vi "UpdateDLLx64.vi"() -> (0 "error out":errorcluster)   [LabVIEW 2017]
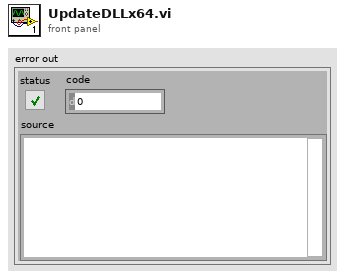
[diagram p1: front panel]
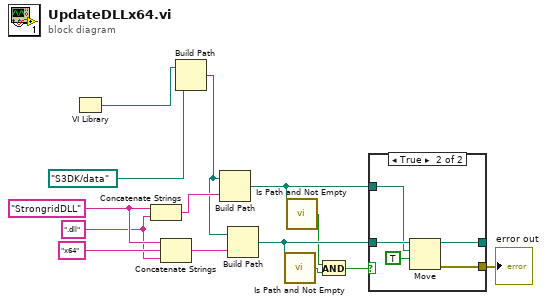
[diagram p0: block diagram]
diagram:
  w12 = ".dll" ("name or relative path")
  w14 = "StrongridDLL" ("name or relative path")
  n1 = VI Library() -> (path=w3:path)
  n2 = Concatenate Strings(w14, w12) -> (w11:string)
  n3 = Concatenate Strings(w14, "x64" ("name or relative path"), w12) -> (w10:string)
  n4 = Build Path(base path=w3, name or relative path=path "S3DK/data") -> (appended path=w1:path)
  n5 = Build Path(base path=w1, name or relative path=w11) -> (appended path=w8:path)
  n6 = Build Path(base path=w1, name or relative path=w10) -> (appended path=w9:path)
  n7 = call <vilib>:"Is Path and Not Empty.vi"("path"=w9) -> ("Is Path and Not Empty?"=w6:bool)  [unwired: 4 in]
  n8 = call <vilib>:"Is Path and Not Empty.vi"("path"=w8) -> ("Is Path and Not Empty?"=w7:bool)  [unwired: 4 in]
  n9 = And(x=w7, y=w6) -> (x .and. y?=w5:bool)
  n10 = case shown="True" w5 {
    tunnel: w9 -> [w15 w20]
    tunnel: w8 -> [_ w19]
    tunnel: [_ w17] -> w4
    tunnel: [w15 w16] -> _
    frame False {
    }
    frame True {
      n11 = Move(source path=w20, 9:TRUE ("overwrite (F)"), 10:w19) -> (error out=w17:errorcluster, 3:w16:path)  [unwired: 2 in, 1 out]
    }
  }
  "error out" <- w4
